vi "Generate Leads.vi"(1 "Leads In":T1) -> (0 "Leads Out":T1)   [LabVIEW 2017]
uses:
  ECG Leads.ctl
  HostCode/HostCode.lvlib
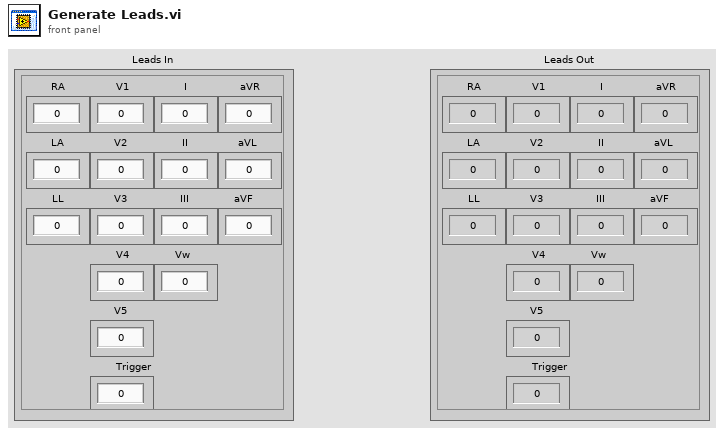
[diagram p1: front panel]
types:
  T1 = typedef "ECG Leads.ctl" = cluster{"RA":i16, "LA":i16, "LL":i16, "V1":i16, "V2":i16, "V3":i16, "V4":i16, "V5":i16, "Trigger":i16, "I":i16, "II":i16, "III":i16, "aVR":i16, "aVL":i16, "aVF":i16, "Vw":i16}
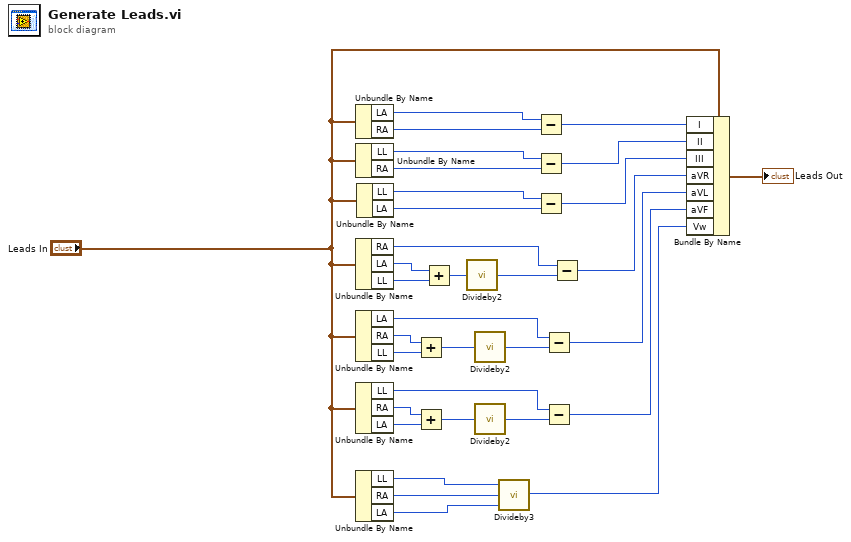
[diagram p0: block diagram]
diagram:
  n1 = Unbundle By Name("Leads In") -> ("LA"=w28:i16, "RA"=w33:i16)
  n2 = Unbundle By Name("Leads In") -> ("LL"=w31:i16, "RA"=w32:i16)
  n3 = Unbundle By Name("Leads In") -> ("RA"=w25:i16, "LA"=w27:i16, "LL"=w26:i16)
  n4 = Unbundle By Name("Leads In") -> ("LA"=w24:i16, "RA"=w22:i16, "LL"=w23:i16)
  n5 = Unbundle By Name("Leads In") -> ("LL"=w19:i16, "RA"=w21:i16, "LA"=w20:i16)
  n6 = Unbundle By Name("Leads In") -> ("LL"=w17:i16, "RA"=w16:i16, "LA"=w15:i16)
  n7 = Unbundle By Name("Leads In") -> ("LL"=w30:i16, "LA"=w29:i16)
  n8 = Add(x=w22, y=w23) -> (x+y=w11:i16)
  n9 = Add(x=w21, y=w20) -> (x+y=w9:i16)
  n10 = Add(x=w27, y=w26) -> (x+y=w13:i16)
  n11 = call "Divideby2.vi"("Input"=w13) -> ("Output"=w12:i16)
  n12 = call "Divideby2.vi"("Input"=w11) -> ("Output"=w10:i16)
  n13 = call "Divideby2.vi"("Input"=w9) -> ("Output"=w8:i16)
  n14 = call "Divideby3.vi"("C"=w15, "B"=w16, "A"=w17) -> ("Divideby3"=w14:i16)
  n15 = Subtract(x=w28, y=w33) -> (x-y=w4:i16)
  n16 = Subtract(x=w31, y=w32) -> (x-y=w3:i16)
  n17 = Subtract(x=w30, y=w29) -> (x-y=w2:i16)
  n18 = Subtract(x=w24, y=w10) -> (x-y=w6:i16)
  n19 = Subtract(x=w19, y=w8) -> (x-y=w5:i16)
  n20 = Subtract(x=w25, y=w12) -> (x-y=w7:i16)
  n21 = Bundle By Name(cluster="Leads In", "I"=w4, "II"=w3, "III"=w2, "aVR"=w7, "aVL"=w6, "aVF"=w5, "Vw"=w14) -> (→"Leads Out":T1)
